vi "Page_Source_Settings_CustVISettings_UpdateDisplay.vi"(8 "error in (no error)":errorcluster, 9 "sourceInclusion":T1, 10 "sourceProperties in":T2[](array[typedef]), 11 "AB_Build in":refnum<class "AB_Build.lvclass">) -> (0 "error out":errorcluster, 1 "Run when opened disabled state":u8, 2 "sourceProperties out":T2[](array[typedef]), 3 "AB_Build out":refnum<class "AB_Build.lvclass">, 5 "AEH disabled state":u8)   [LabVIEW 2020, in "AB_Build.lvclass"]
uses:
  <vilib>/AppBuilder/AB_Classes/Build/AB_Build.lvclass
  <vilib>/AppBuilder/AB_Source_Properties.ctl
  <vilib>/AppBuilder/AB_Source_Property_Type.ctl
  <vilib>/AppBuilder/AB_Source_Inclusion.ctl
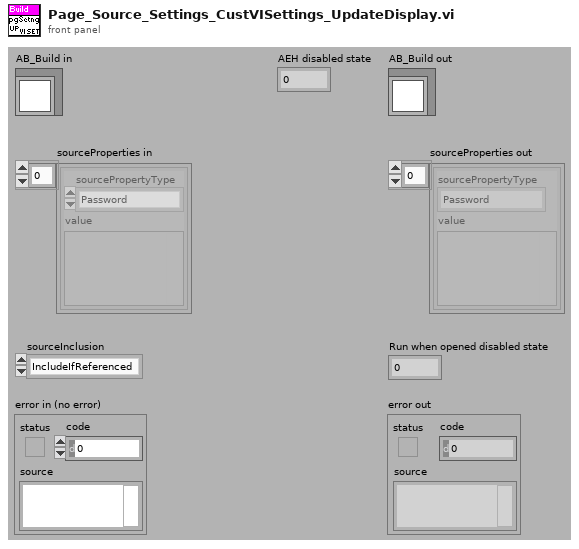
[diagram p1: front panel]
types:
  T1 = typedef "AB_Source_Inclusion.ctl" = enum16{"IncludeIfReferenced", "Include", "Exclude", "TopLevel"}
  T2 = typedef "AB_Source_Properties.ctl" = cluster{"sourcePropertyType":T3, "value":variant}
  T3 = typedef "AB_Source_Property_Type.ctl" = enum16{"Remove block diagram", "Remove front panel", "Password", "Window has title bar", "Show menu bar", "Show vertical scroll bar", "Show horizontal scroll bar", "Show toolbar", "Show Abort button", "Show fp when called", "Window behavior", "Allow user to close window", "Window run-time position", "Run when opened", "Allow debugging", "Auto error handling", "Generate guard code", "Use stack variables", "Expression folding", "Integer only", "Inline subVI"}
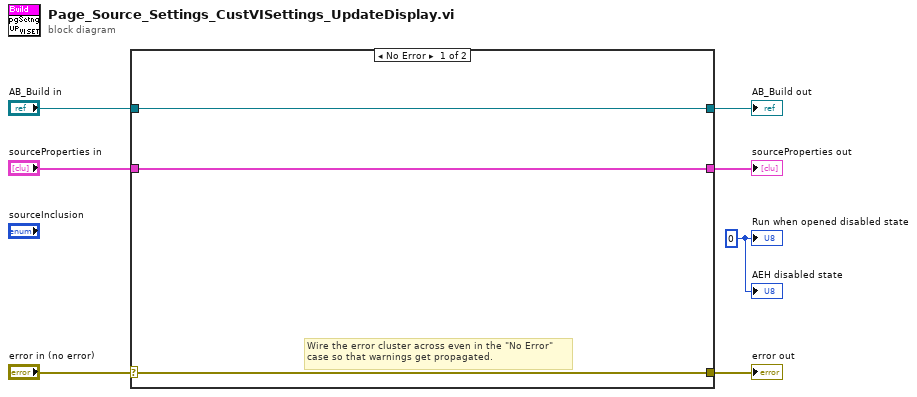
[diagram p0: block diagram]
diagram:
  w1 = u8 0 ("Run when opened disabled state")
  n1 = case shown="No Error" "error in (no error)" {
    selector: "error in (no error)" -> [w9 w13]
    tunnel: [w9 w13] -> w6
    tunnel: [w10 w12] -> w4
    tunnel: "AB_Build in" -> [w10 w12]
    tunnel: "sourceProperties in" -> [w8 w11]
    tunnel: [w8 w11] -> w2
    frame No Error {
      # "Wire the error cluster across even in the \"No Error\"\ncase so that warnings get propagated."
    }
    frame Error {
    }
  }
  "error out" <- w6
  "AB_Build out" <- w4
  "sourceProperties out" <- w2
  "Run when opened disabled state" <- w1
  "AEH disabled state" <- w1
